vi "Convert Version String to Version Descriptor.vi"(8 "Error In":errorcluster, 11 "Version Number (String)":string) -> (0 "Error Out":errorcluster, 3 "Version Description":T1={"Major Version Number"=0, "Minor Version Number"=0, "Revision Number"=0, "Version Type"=enum."release", "a/b/rc/ Version Number"=0})   [LabVIEW 2021, in "Strings.lvlib"]
uses:
  Strings.lvlib
  Utilities/Version Type.ctl
  Utilities/Version Description.ctl
  Utilities/Utilities.lvlib
panel:
  out "a/b/rc/ Version Number":i32
  out "Version Type":T2=enum."release"
  out "Revision Number":i32
  out "Major Version Number":i32
  out "Indices":i32[](array[numeric])
  out "Tokens":string[](array[string])
  out "Minor Version Number":i32
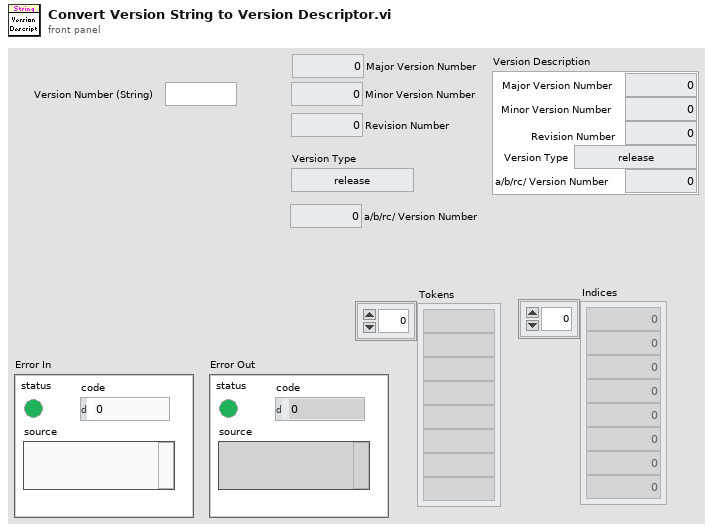
[diagram p1: front panel]
types:
  T1 = typedef "Utilities.lvlib/Version Description.ctl" = cluster{"Major Version Number":i32, "Minor Version Number":i32, "Revision Number":i32, "Version Type":T2, "a/b/rc/ Version Number":i32}
  T2 = typedef "Utilities.lvlib/Version Type.ctl" = enum16{"alpha", "beta", "release candidate", "release"}
  T3 = enum16{"major", "minor", "revision", "type number"}
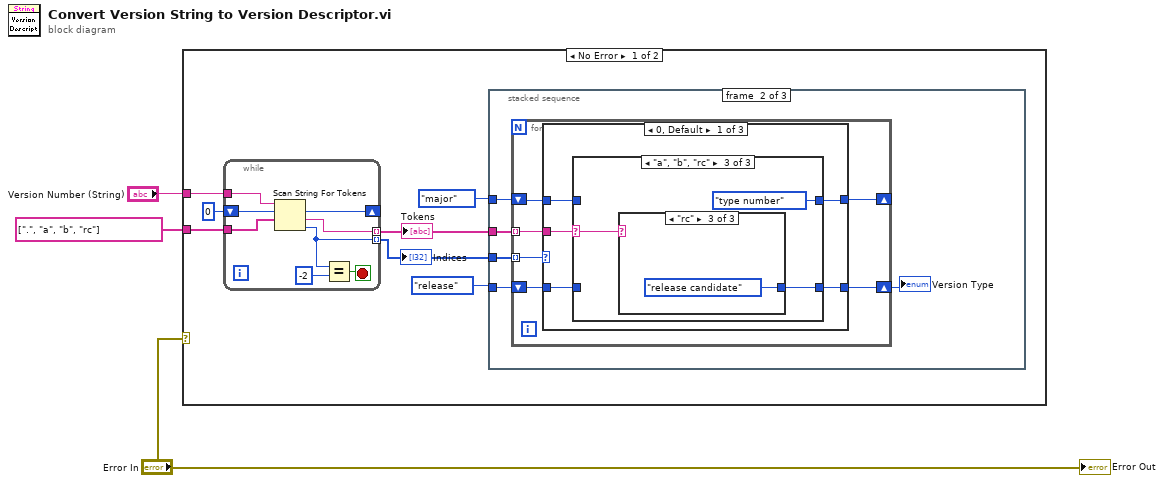
[diagram p0: block diagram]
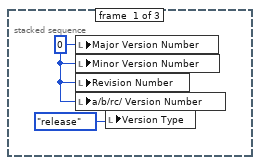
[diagram p2: hidden frame]
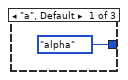
[diagram p5: hidden frame]
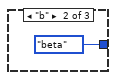
[diagram p6: hidden frame]
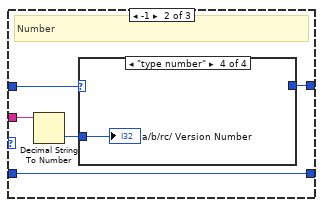
[diagram p7: hidden frame]
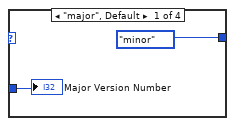
[diagram p8: hidden frame]
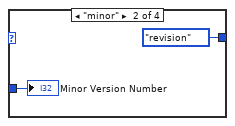
[diagram p9: hidden frame]
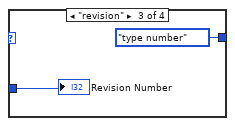
[diagram p10: hidden frame]
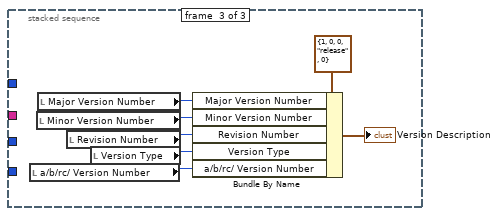
[diagram p12: hidden frame]
diagram:
  n1 = case shown="No Error" "Error In" {
    tunnel: "Version Number (String)" -> [w10 _]
    tunnel: string[] [".", "a", "b", "rc"] ("operators (none)") -> [w9 _]
    frame No Error {
      n2 = while {
        tunnel: w10 -> [w67]
        tunnel: w9 -> [w66]
        shift-right: [w65] -> _
        shift-left: 0 ("offset past token") -> [w60]
        tunnel: [w64] -> w7 mode=indexing
        tunnel: [w63] -> w6 mode=indexing
        stop <- w61 stop-if-true
        n3 = Scan String For Tokens(7:w66, 8:w60, 9:w67) -> (0:w63:i32, 1:w64:string, 2:w65:i32)  [unwired: 3 in, 1 out]
        n4 = Equal?(x=w63, y=-2) -> (x = y?=w61:bool)
      }
      "Tokens" <- w7
      "Indices" <- w6
      n5 = stacked-sequence {
        tunnel: w7 -> [_ w17 _]
        tunnel: w6 -> [_ w16 _]
        tunnel: T3."major" -> [_ w15 _]
        tunnel: Version_Type."release" ("Version Type") -> [_ w14 _]
        frame #0 {
          w12 = 0 ("Major Version Number")
          n6 = local write "Major Version Number"(w12) -> ()
          n7 = local write "Minor Version Number"(w12) -> ()
          n8 = local write "Revision Number"(w12) -> ()
          n9 = local write "a/b/rc/ Version Number"(w12) -> ()
          n10 = local write "Version Type"(Version_Type."release" ("Version Type")) -> ()
        }
        frame #1 {
          n11 = for {
            tunnel: w17 -> [w22] mode=indexing
            tunnel: w16 -> [w23] mode=indexing
            shift-right: [w20] -> _
            shift-left: w15 -> [w21]
            shift-right: [w18] -> w13
            shift-left: w14 -> [w19]
            n12 = case shown="0, Default" w23 {
              tunnel: w22 -> [w28 w42 _]
              tunnel: w21 -> [w25 w43 w52]
              tunnel: [w24 w40 w52] -> w20
              tunnel: w19 -> [w27 w39 w51]
              tunnel: [w26 w39 w51] -> w18
              frame 0, Default {
                n13 = case shown="\"a\", \"b\", \"rc\"" w28 {
                  selector: w28 -> [_ _ w35]
                  tunnel: w27 -> [w30 w32 _]
                  tunnel: [w30 w32 w34] -> w26
                  tunnel: w25 -> [w29 w31 _]
                  tunnel: [w29 w31 T3."type number"] -> w24
                  frame "", Default {
                  }
                  frame "." {
                  }
                  frame "a", "b", "rc" {
                    n14 = case shown="\"rc\"" w35 {
                      tunnel: [Version_Type."alpha" ("Version Type") Version_Type."beta" ("Version Type") Version_Type."release candidate" ("Version Type")] -> w34
                      frame "a", Default {
                      }
                      frame "b" {
                      }
                      frame "rc" {
                      }
                    }
                  }
                }
              }
              frame -1 {
                # "Number"
                n15 = Decimal String To Number(string=w42) -> (number=w41:i32)  [unwired: 2 in, 1 out]
                n16 = case shown="\"type number\"" w43 {
                  tunnel: w41 -> [w45 w47 w49 w50]
                  tunnel: [T3."minor" T3."revision" T3."type number" _] -> w40
                  frame "major", Default {
                    "Major Version Number" <- w45
                  }
                  frame "minor" {
                    "Minor Version Number" <- w47
                  }
                  frame "revision" {
                    "Revision Number" <- w49
                  }
                  frame "type number" {
                    "a/b/rc/ Version Number" <- w50
                  }
                }
              }
              frame -2 {
              }
            }
          }
          "Version Type" <- w13
        }
        frame #2 {
          n17 = local read "a/b/rc/ Version Number"() -> (w55:i32)
          n18 = local read "Minor Version Number"() -> (w58:i32)
          n19 = local read "Major Version Number"() -> (w59:i32)
          n20 = local read "Revision Number"() -> (w57:i32)
          n21 = local read "Version Type"() -> (w56:T2)
          n22 = Bundle By Name(cluster=T1 {"Major Version Number"=1, "Minor Version Number"=0, "Revision Number"=0, "Version Type"=enum."release", "a/b/rc/ Version Number"=0} ("Version Description"), "Major Version Number"=w59, "Minor Version Number"=w58, "Revision Number"=w57, "Version Type"=w56, "a/b/rc/ Version Number"=w55) -> (→"Version Description":T1)
        }
      }
    }
    frame Error {
    }
  }
  "Error Out" <- "Error In"
